vi "S2C_SaveReport.vi"(8 "Error In":errorcluster, 11 "Result":string) -> (0 "Error Out":errorcluster)   [LabVIEW 2015]
doc: "If enabled, saves the test report to the local drive."
uses:
  Globals/S2C_Globals.vi
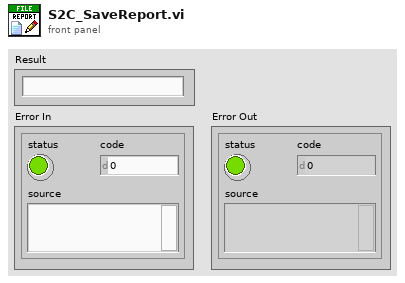
[diagram p1: front panel]
types:
  T1 = enum16{"open", "replace", "create", "open or create", "replace or create", "replace or create with confirmation"}
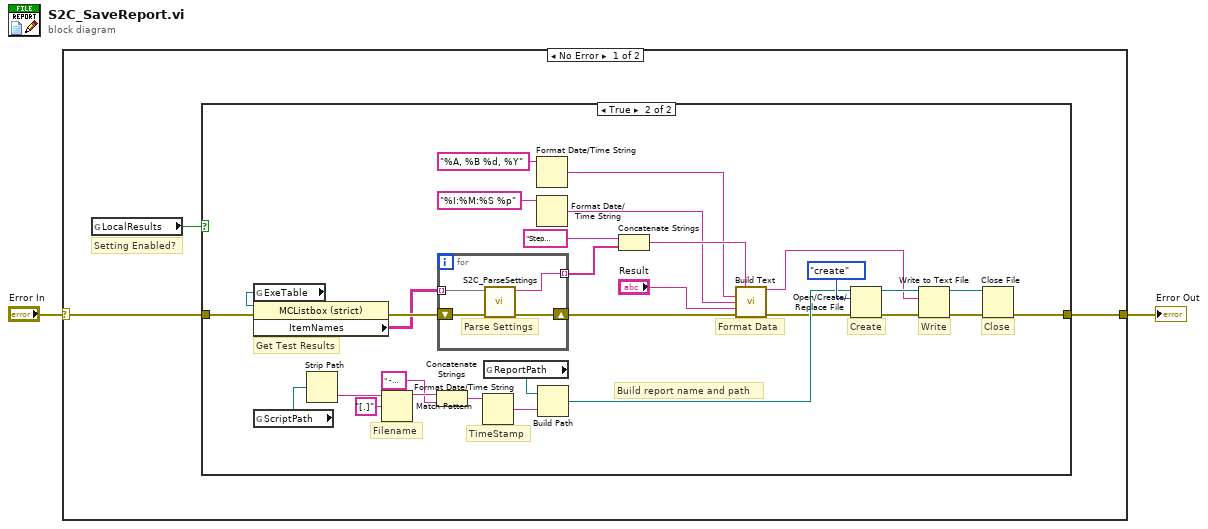
[diagram p0: block diagram]
diagram:
  n1 = case shown="No Error" "Error In" {
    selector: "Error In" -> [w5 w41]
    tunnel: [w4 w41] -> w1
    frame No Error {
      # "Setting Enabled?"
      n2 = global read "S2C_Globals.vi" "LocalResults"() -> (w3:bool)
      n3 = case shown="True" w3 {
        tunnel: w5 -> [w6 w35]
        tunnel: [w6 w18] -> w4
        frame False {
          # "Local report creation is not enabled"
        }
        frame True {
          # "TimeStamp"
          # "Filename"
          # "Build report name and path"
          # "Format Data"
          # "Close"
          # "Write"
          # "Create"
          # "Get Test Results"
          n4 = global read "S2C_Globals.vi" "ExeTable"() -> (w36:refnum<vi>)
          n5 = property class="MCListbox (strict)"(reference=w36, error in=w35) -> (error out=w16:errorcluster, "ItemNames"=w14:string[][])  [unwired: 1 out]
          n6 = global read "S2C_Globals.vi" "ScriptPath"() -> (w11:path)
          n7 = Strip Path(path=w11) -> (name=w12:string)  [unwired: 1 out]
          n8 = Match Pattern(string=w12, regular expression="[.]") -> (before substring=w10:string)  [unwired: 1 in, 3 out]
          n9 = Concatenate Strings(w10, " - [%m_%d_%Y - %I_%M_%S %p].txt" ("time format string (%c)")) -> (w9:string)
          n10 = for {
            tunnel: [w37] -> w34 mode=indexing
            shift-right: [w38] -> w15
            shift-left: w16 -> [w40]
            tunnel: w14 -> [w39] mode=indexing
            # "Parse Settings"
            n11 = call "S2C_ParseSettings.vi"("Error In"=w40, "Table Data"=w39) -> ("Error Out"=w38:errorcluster, "Result"=w37:string)  [unwired: 8 in]
          }
          n12 = Format Date/Time String(time format string (%c)=w9) -> (date/time string=w26:string)  [unwired: 2 in]
          n13 = global read "S2C_Globals.vi" "ReportPath"() -> (w17:path)
          n14 = Format Date/Time String(time format string (%c)="%A, %B %d, %Y") -> (date/time string=w30:string)  [unwired: 2 in]
          n15 = Format Date/Time String(time format string (%c)="%I:%M:%S %p") -> (date/time string=w29:string)  [unwired: 2 in]
          n16 = Build Path(base path=w17, name or relative path=w26) -> (appended path=w25:path)
          n17 = Concatenate Strings("Step Name\tTest Parameter\tLL Comp\tLow Limit\tMeasurement\tHigh Limit\tHL Comp\tTime\tResult\n", w34) -> (w31:string)
          n18 = call "Build Text"("Data"=w31, "Date"=w30, "Time"=w29, "Result"="Result", "error in (no error)"=w15) -> ("Result"=w21:string, "error out"=w24:errorcluster)  [unwired: 9 in]
          n19 = Open/Create/Replace File(file path (use dialog)=w25, error in=w24, operation (0:open)=T1."create") -> (refnum out=w22:refnum<file>, error out=w23:errorcluster)  [unwired: 3 in, 1 out]
          n20 = Write to Text File(file (use dialog)=w22, text=w21, error in=w23) -> (refnum out=w19:refnum<file>, error out=w20:errorcluster)  [unwired: 1 in, 1 out]
          n21 = Close File(refnum=w19, error in=w20) -> (error out=w18:errorcluster)  [unwired: 1 out]
        }
      }
    }
    frame Error {
    }
  }
  "Error Out" <- w1
